vi "aryth_block.vi"(2 "Control":T3, 3 "B":T4, 4 "A":T5) -> (0 "Flags":T1, 1 "Result":T2)   [LabVIEW 2013]
panel:
  # "R1"
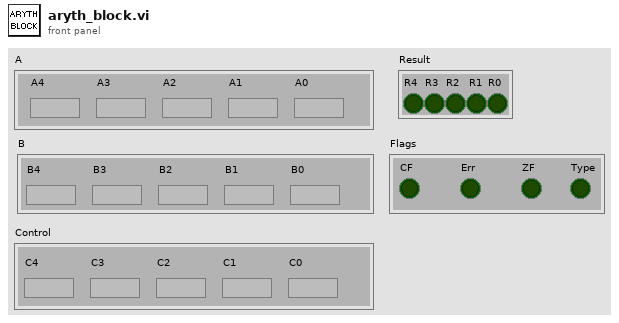
[diagram p1: front panel]
types:
  T1 = cluster{"CF":bool, "Err":bool, "ZF":bool, "Type":bool}
  T2 = cluster{"R4":bool, "R3":bool, "R2":bool, bool, "R0":bool}
  T3 = cluster{"C4":bool, "C3":bool, "C2":bool, "C1":bool, "C0":bool}
  T4 = cluster{"B4":bool, "B3":bool, "B2":bool, "B1":bool, "B0":bool}
  T5 = cluster{"A4":bool, "A3":bool, "A2":bool, "A1":bool, "A0":bool}
  T6 = cluster{"Result":cluster{"R4":bool, "R3":bool, "R2":bool, bool, "R0":bool}, "Result":cluster{"R4":bool, "R3":bool, "R2":bool, bool, "R0":bool}, "Result":cluster{"R4":bool, "R3":bool, "R2":bool, bool, "R0":bool}}
  T7 = cluster{"Flags":cluster{"CF":bool, "Err":bool, "ZF":bool, "Type":bool}, "Flags":cluster{"CF":bool, "Err":bool, "ZF":bool, "Type":bool}, "Flags":cluster{"CF":bool, "Err":bool, "ZF":bool, "Type":bool}}
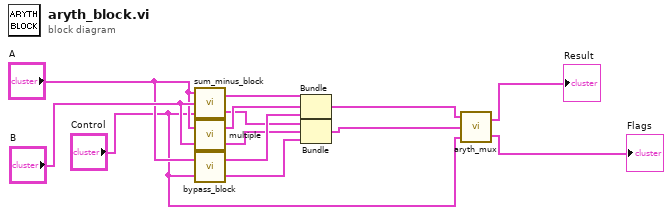
[diagram p0: block diagram]
diagram:
  n1 = call "sum_minus_block.vi"("Control"="Control", "B"="B", "A"="A") -> ("Flags"=w5:T1, "Result"=w8:T2)
  n2 = call "multiple.vi"("B"="B", "A"="A") -> ("Flags"=w4:T1, "Result"=w7:T2)
  n3 = call "bypass_block.vi"("Control"="Control", "A"="A") -> ("Flags"=w3:T1, "Result"=w6:T2)
  n4 = Bundle("Result"=w8, "Result"=w7, "Result"=w6) -> (w1:T6)  [unwired: 1 in]
  n5 = Bundle("Flags"=w5, "Flags"=w4, "Flags"=w3) -> (w2:T7)  [unwired: 1 in]
  n6 = call "aryth_mux.vi"("Control"="Control", "Flags_input"=w2, "Results_input"=w1) -> ("Flags"=→"Flags":T1, "Result"=→"Result":T2)
